vi "labview_camerasleft_hand_cameraimage_Server.vi"() -> ()   [LabVIEW 2013]
doc: "Template server that runs individual ros topics, services, etc. This is cloned for each topic being run."
uses:
  SubVIs/_ROSControl.ctl
  SubVIs/_ROSDirection.ctl
  _ROSDefinition.vi
panel:
  out "Init Count":i32
  out "queue":string
  out "Connected":bool
  out "str to write":string
  out "Status":T1(ring) caption="Connected?"
  out "Specs":T3={"Server"="", "Node"="/labview", "Server Port"=5000, "URI (Subsc)"="", "Direction"=enum."Node"}
  out "Service Reply":string
  out "unregister":string="<?xml version='1.0'?>\n<methodResponse>\n<params>\n<param>\n<value><array><data>\n<value><int>1</int></value>\n<value><string>Registered [/labview] as publisher of [/robot/head/command_head_nod]</string></value>\n<value><array><data>\n<value><string>http://tuftsBaxter.local:56995/</string></value>\n</data></array></value>\n</data></array></value>\n</param>\n</params>\n</methodResponse>\n"
  out "Requests":T4(array[cluster])
  out "Last Reply":string
  in  "stop":bool
  out "error out":errorcluster
  out "Connections":T5(array[cluster])
  in  "Baxter":T6
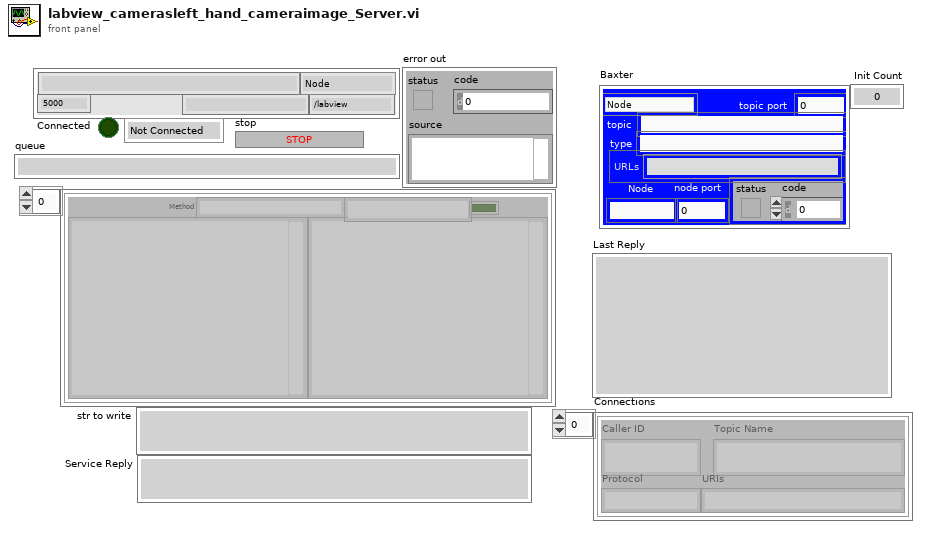
[diagram p1: front panel]
types:
  T1 = enum16{"Not Connected", "Registered", "Connected"}
  T2 = typedef "_ROSDirection.ctl" = enum16{"Node", "Publisher", "Subscriber", "Service Client"}
  T3 = cluster{"Server":string, "Node":string, "Server Port":u32, "URI (Subsc)":string, "Direction":T2}
  T4 = cluster{"First":string, "Second":string, "Method":string, "success":bool, "Dir1":string, "Dir2":string, "time":string}[]
  T5 = cluster{"Caller ID":string, "Topic Name":string, "Protocol":string, "URIs":string}[]
  T6 = typedef "_ROSControl.ctl" = cluster{"topic port":u16, "Node":string, "topic":string, "type":string, "node port":u32, "error ":errorcluster, "Direction":T2, "APIs":string[]}
  T7 = cluster{"data out":string, "data out 2":string, "data out 3":string, "Success?":bool, "data out 4":string, "data out 5":string, "time":string}[]
  T8 = cluster{"Code":i32, "Status Message":string, "APIs":string[]}
  T9 = cluster{"Server":string, "Node":string, "Server Port":u32, "URI (Subsc)":string, "connection":refnum<k5>, "Direction":T2}
  T10 = cluster{"Caller ID":string, "Topic Name":string, "Protocol":string, "URIs":string}
  T11 = cluster{string, "data out":string, "Node":string, bool, string, string, "Current Time":string}
  T12 = cluster{string, string, string, bool, string, string, "Current Time":string}
  T13 = cluster{"Protocol":string, "Code":i32, "IP":string, "Port":i32}
  T14 = cluster{"Node":string, "topic":string, "topic":string, "topic":string}
  T15 = cluster{"Code":i8, "statusMessage":string, "APIs":string[]}
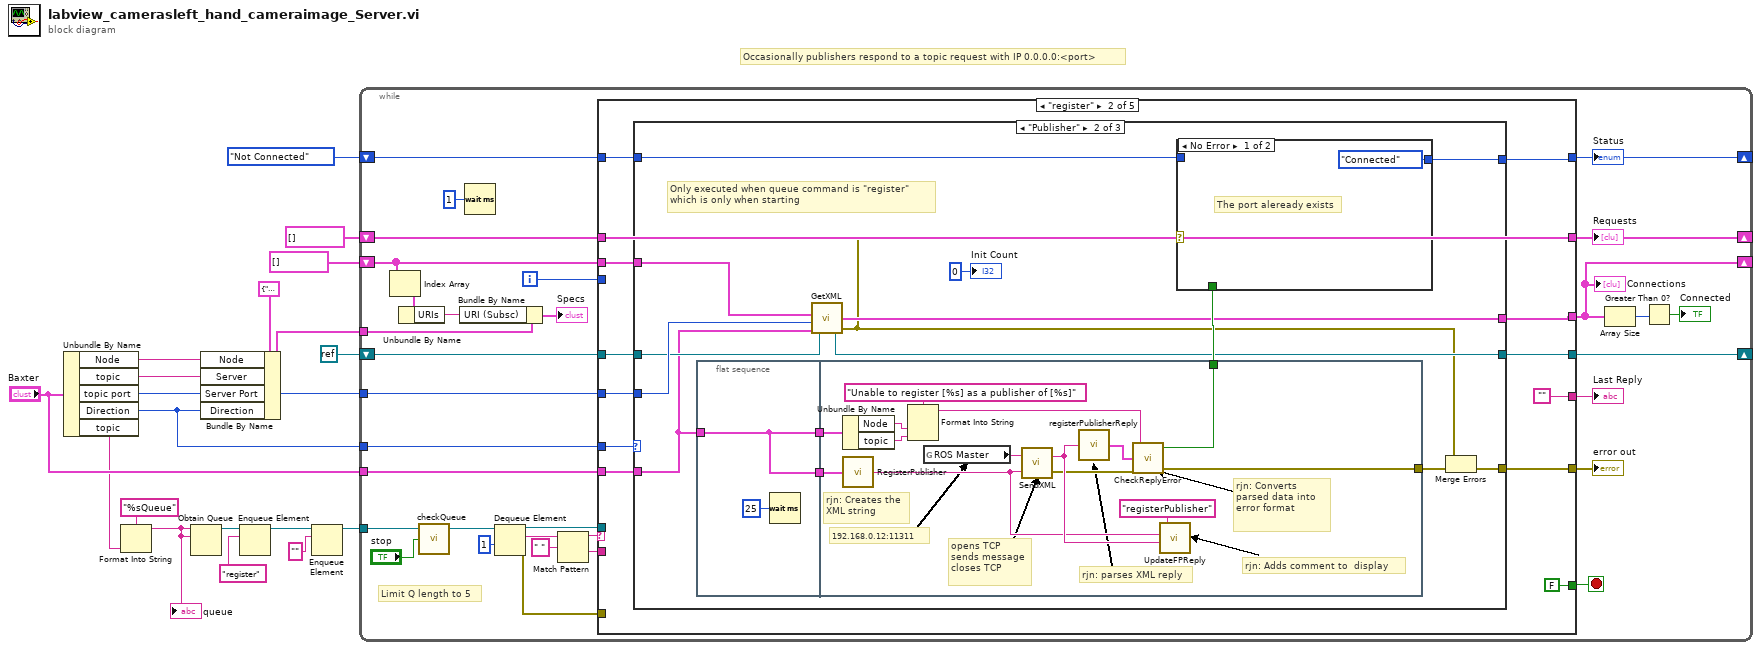
[diagram p0: block diagram]
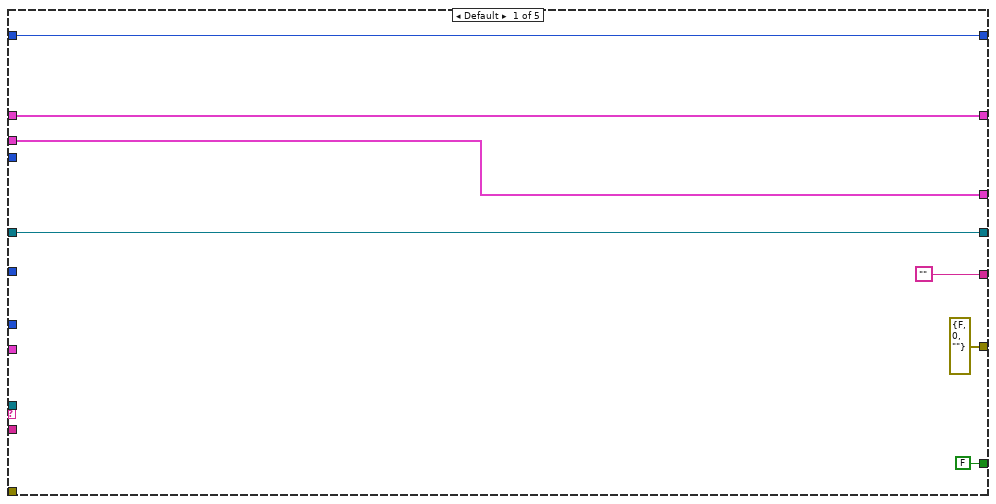
[diagram p2: hidden frame]
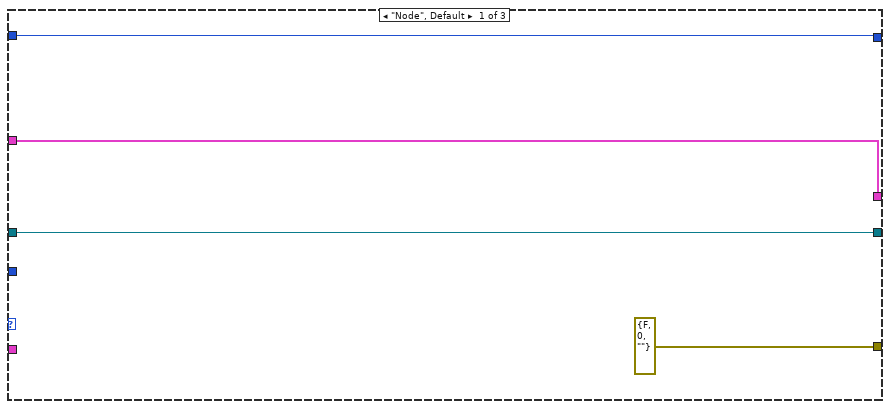
[diagram p3: hidden frame]
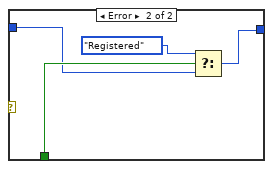
[diagram p4: hidden frame]
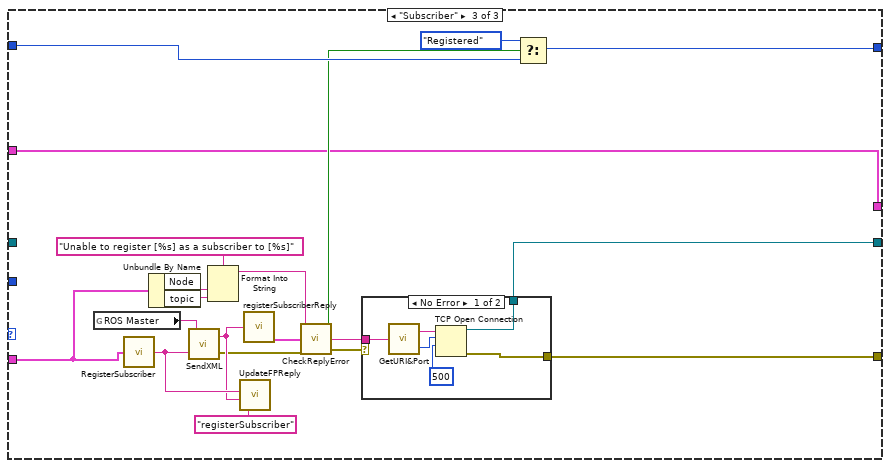
[diagram p5: hidden frame]
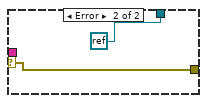
[diagram p6: hidden frame]
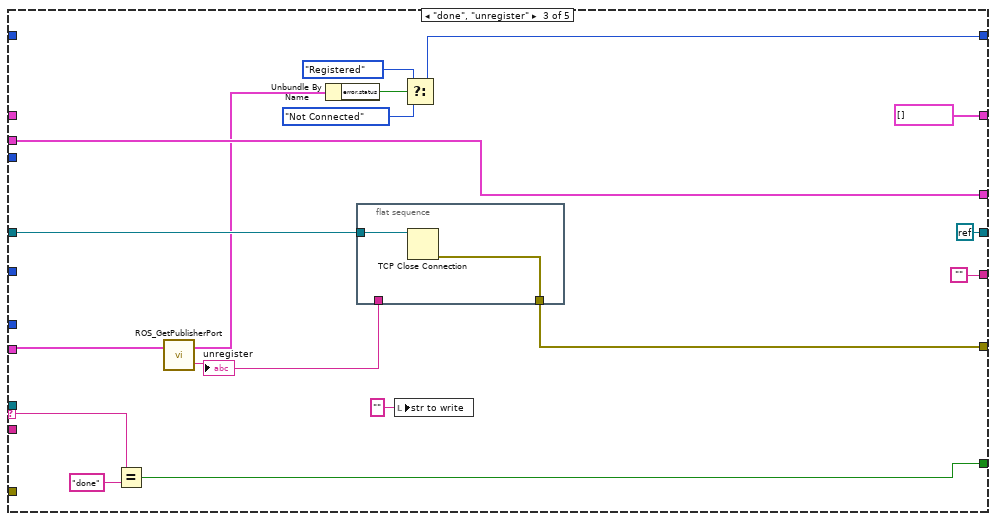
[diagram p7: hidden frame]
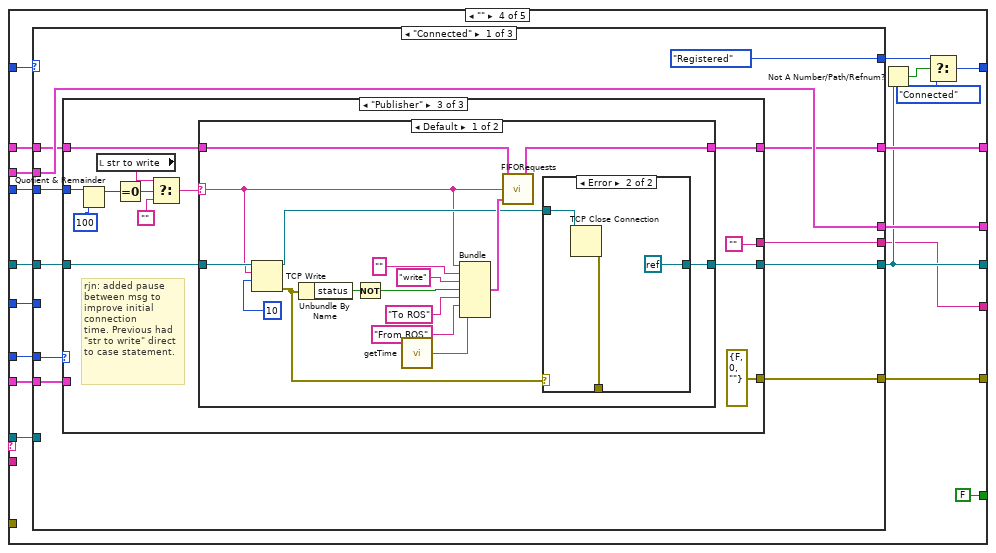
[diagram p8: hidden frame]
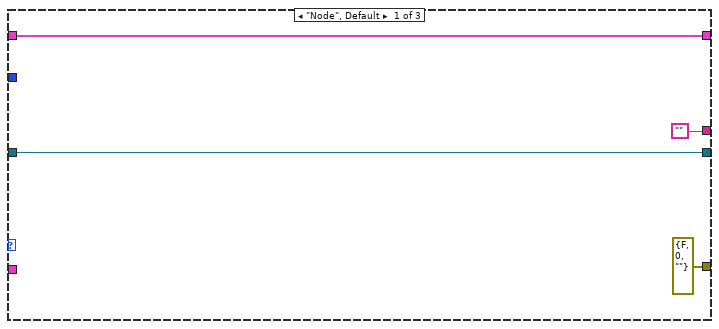
[diagram p9: hidden frame]
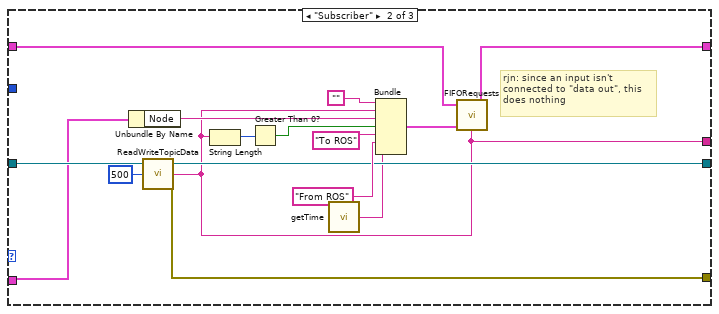
[diagram p10: hidden frame]
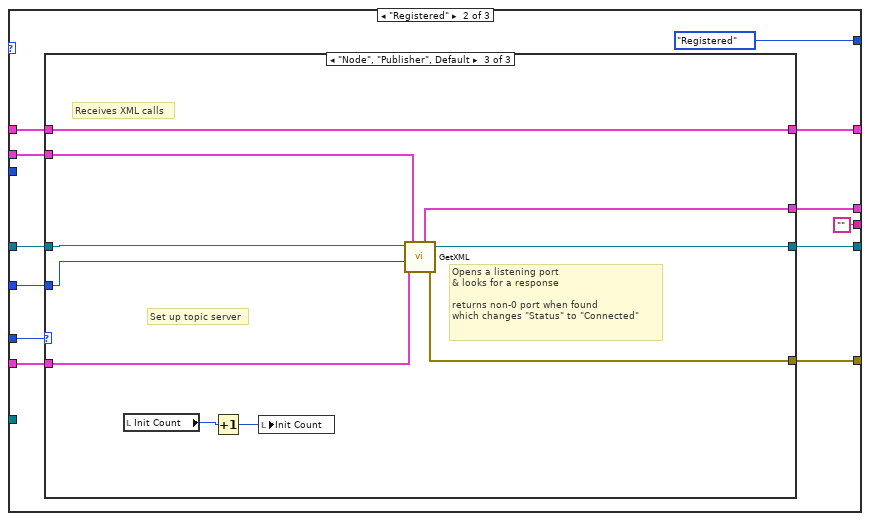
[diagram p13: hidden frame]
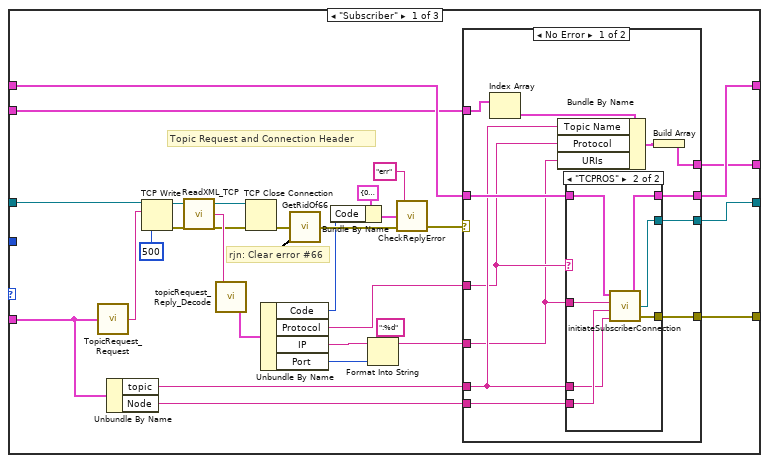
[diagram p14: hidden frame]
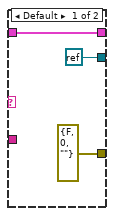
[diagram p15: hidden frame]
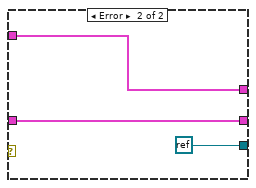
[diagram p16: hidden frame]
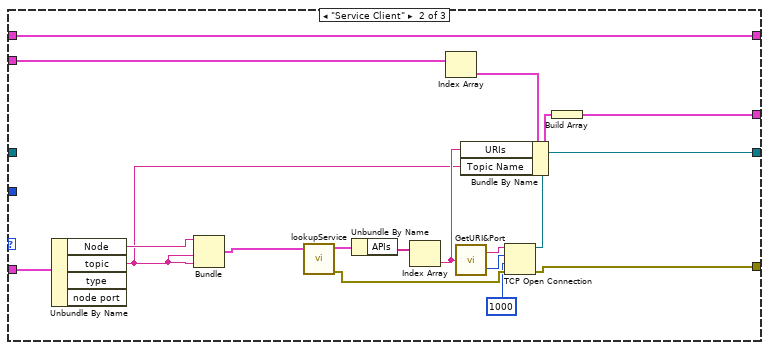
[diagram p17: hidden frame]
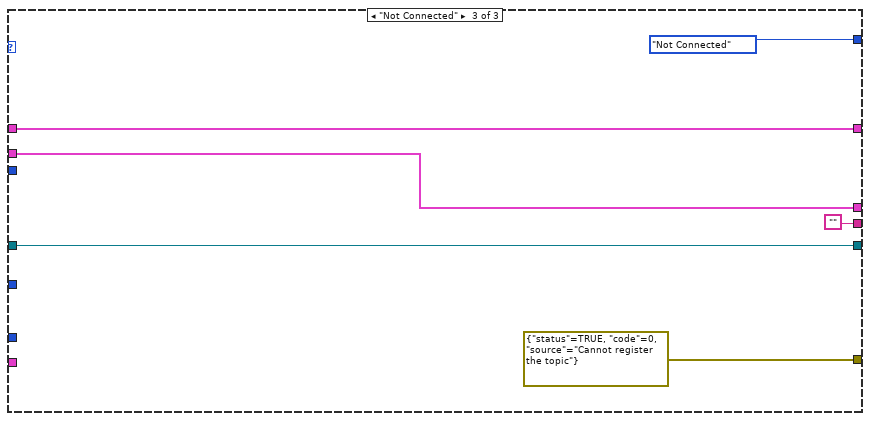
[diagram p18: hidden frame]
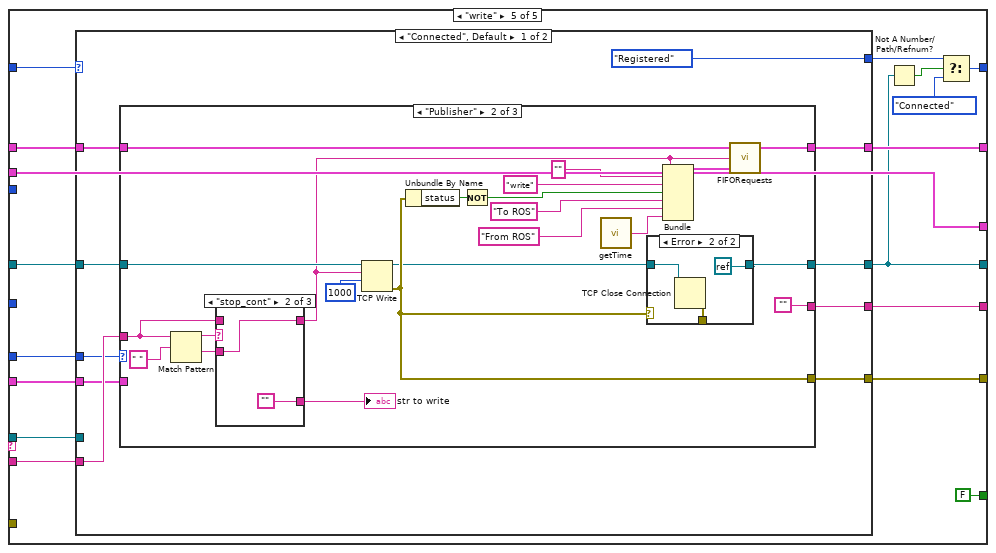
[diagram p19: hidden frame]
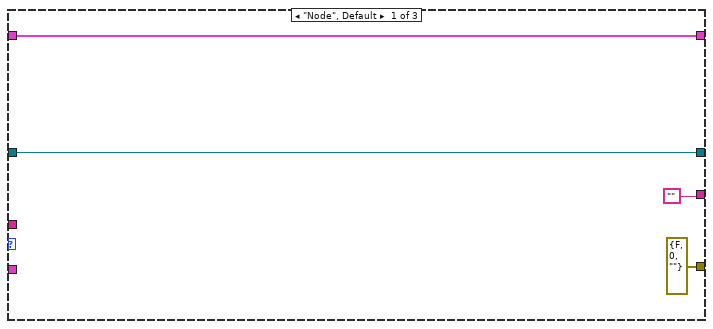
[diagram p20: hidden frame]
diagram:
  # "Occasionally publishers respond to a topic request with IP 0.0.0.0:<port>"
  n1 = Unbundle By Name("Baxter") -> ("Node"=w4:string, "topic"=w3:string, "topic port"=w1:u16, "Direction"=w2:T2, "topic"=w9:string)
  n2 = Format Into String(format string="%sQueue", w9) -> (resulting string=w18:string)  [unwired: 2 in, 1 out]
  "queue" <- w18
  n3 = Obtain Queue(name (unnamed)=w18, element data type=w18) -> (queue out=w12:refnum<queue>)  [unwired: 3 in, 2 out]
  n4 = Bundle By Name(cluster=T3 {"Server"="", "Node"="/labview", "Server Port"=5000, "URI (Subsc)"="", "Direction"=enum."Node"} ("Specs"), "Node"=w4, "Server"=w3, "Server Port"=w1, "Direction"=w2) -> (w10:T3)
  n5 = Enqueue Element(queue=w12, element="register") -> (queue out=w7:refnum<queue>)  [unwired: 2 in, 2 out]
  n6 = Enqueue Element(queue=w7, element="") -> (queue out=w6:refnum<queue>)  [unwired: 2 in, 2 out]
  n7 = while {
    tunnel: w1 -> [w51]
    shift-right: [w25] -> _
    shift-left: T5 [] ("Connections") -> [w34]
    shift-right: [w40] -> _
    shift-left: refnum<k0> refnum -> [w49]
    tunnel: w2 -> [w50]
    tunnel: "Baxter" -> [w48]
    shift-right: [w41] -> _
    shift-left: T7 [] ("Requests In") -> [w42]
    shift-right: [w37] -> _
    shift-left: T1."Not Connected" ("Status") -> [w38]
    tunnel: w10 -> [w32]
    tunnel: w6 -> [w26]
    i -> [w20]
    stop <- w39 stop-if-true
    # "Limit Q length to 5"
    n8 = Index Array(array=w34) -> (element=w33:T10)  [unwired: 1 in]
    n9 = Unbundle By Name(w33) -> ("URIs"=w31:string)
    n10 = call "checkQueue.vi"("stop"="stop", "queue in"=w26) -> ("queue out"=w28:refnum<queue>)  [unwired: 3 in]
    n11 = Bundle By Name(cluster=w32, "URI (Subsc)"=w31) -> (→"Specs":T3)
    n12 = Wait (ms)(milliseconds to wait=u32 1 ("millisecond multiple")) -> ()  [unwired: 1 out]
    n13 = Dequeue Element(queue=w28, timeout in ms (-1)=1) -> (queue out=w29:refnum<queue>, element=w46:string, error out=w22:errorcluster)  [unwired: 1 in, 1 out]
    n14 = Match Pattern(string=w46, regular expression=" ") -> (before substring=w44:string, after substring=w43:string)  [unwired: 1 in, 2 out]
    n15 = case shown="\"register\"" w44 {
      selector: w44 -> [_ _ w145 _ _]
      tunnel: w51 -> [_ w70 _ w177 _]
      tunnel: w34 -> [w58 w62 w155 w176 w361]
      tunnel: [w58 w61 w155 w175 w361] -> w25
      tunnel: w50 -> [_ w71 _ w174 w353]
      tunnel: [w57 w67 refnum<k0> refnum w168 w354] -> w40
      tunnel: w49 -> [w57 w66 w156 w169 w360]
      tunnel: w48 -> [_ w69 w154 w173 w351]
      tunnel: w43 -> [_ _ _ _ w358]
      tunnel: [FALSE FALSE w143 FALSE FALSE] -> w39
      tunnel: [errorcluster {"status"=FALSE, "code"=0, "source"=""} ("error out") w68 w148 w170 w355] -> w36
      tunnel: w42 -> [w56 w65 _ w172 w357]
      tunnel: [w56 w65 T7 [] ("Requests Out") w171 w356] -> w41
      tunnel: w38 -> [w55 w64 _ w162 w359]
      tunnel: [w55 w63 w150 w163 w346] -> w37
      tunnel: ["" "" "" w167 w352] -> w35
      tunnel: w29 -> [_ _ _ w166 w350]
      tunnel: w22 -> [_ _ _ _ _]
      tunnel: w20 -> [_ _ _ w159 _]
      frame Default {
      }
      frame "register" {
        n16 = case shown="\"Publisher\"" w71 {
          tunnel: w70 -> [_ w85 _]
          tunnel: w69 -> [_ w82 w122]
          tunnel: [errorcluster {"status"=FALSE, "code"=0, "source"=""} ("error IO") w80 w119] -> w68
          tunnel: [w75 w83 w120] -> w67
          tunnel: w66 -> [w75 w84 _]
          tunnel: w64 -> [w74 w89 w115]
          tunnel: [w74 w88 w113] -> w63
          tunnel: w62 -> [w73 w87 w112]
          tunnel: [w73 w86 w112] -> w61
          frame "Node", Default {
          }
          frame "Publisher" {
            # "Only executed when queue command is \"register\"\nwhich is only when starting"
            n17 = flat-sequence {
              tunnel: w82 -> [w91]
              tunnel: [w91] -> w78
              tunnel: [w91] -> w76
              tunnel: [w96] -> w90
              tunnel: [w94] -> w81
              tunnel: w78 -> [w95]
              tunnel: w76 -> [w93]
              frame #0 {
                n18 = Wait (ms)(milliseconds to wait=u32 25) -> ()  [unwired: 1 out]
              }
              frame #1 {
                # "rjn: Adds comment to  display"
                # "rjn: Converts parsed data into\nerror format"
                # "rjn: parses XML reply"
                # "192.168.0.12:11311"
                # "opens TCP\nsends message\ncloses TCP"
                # "rjn: Creates the \nXML string"
                n19 = Unbundle By Name(w95) -> ("Node"=w102:string, "topic"=w101:string)
                n20 = call "RegisterPublisher.vi"("ROS"=w93) -> ("XML"=w100:string)
                n21 = Format Into String(format string="Unable to register [%s] as a publisher of [%s]", w102, w101) -> (resulting string=w98:string)  [unwired: 2 in, 1 out]
                n22 = global read "_ROSDefinition.vi" "ROS Master"() -> (w106:string)
                n23 = call "SendXML.vi"("Send"=w100, "URI in"=w106) -> ("error out"=w97:errorcluster, "Reply"=w105:string)
                n24 = call "registerPublisherReply.vi"("Response"=w105) -> ("Response"=w99:T8)
                n25 = call "CheckReplyError.vi"("error in"=w97, "Response"=w99, "Error String"=w98) -> ("error out"=w94:errorcluster, "Registered?"=w96:bool)  [unwired: 1 out]
                n26 = call "UpdateFPReply.vi"("Reply"=w105, "Sent"=w100, "method"="registerPublisher") -> ()  [unwired: 3 in]
              }
            }
            n27 = call "GetXML.vi"("Baxter"=w82, "topic port"=w85, "Connections"=w87, "connection ID in"=w84) -> ("error IO"=w79:errorcluster, "Subscribers"=w86:T5, "connection ID out"=w83:refnum<k5>)
            n28 = case shown="No Error" w79 {
              tunnel: w90 -> [_ w111]
              tunnel: w89 -> [_ w110]
              tunnel: [T1."Connected" ("f") w108] -> w88
              frame No Error {
                # "The port aleready exists"
              }
              frame Error {
                n29 = Select(t=T1."Registered", s=w111, f=w110) -> (s? t:f=w108:T1)
              }
            }
            n30 = Merge Errors(w79, w81) -> (w80:errorcluster)
            "Init Count" <- 0
          }
          frame "Subscriber" {
            n31 = global read "_ROSDefinition.vi" "ROS Master"() -> (w131:string)
            n32 = call "RegisterSubscriber.vi"("ROS"=w122) -> ("XML"=w129:string)
            n33 = Unbundle By Name(w122) -> ("Node"=w126:string, "topic"=w125:string)
            n34 = call "SendXML.vi"("Send"=w129, "URI in"=w131) -> ("error out"=w118:errorcluster, "Reply"=w128:string)
            n35 = Format Into String(format string="Unable to register [%s] as a subscriber to [%s]", w126, w125) -> (resulting string=w123:string)  [unwired: 2 in, 1 out]
            n36 = call "UpdateFPReply.vi"("Reply"=w128, "Sent"=w129, "method"="registerSubscriber") -> ()  [unwired: 3 in]
            n37 = call "registerSubscriberReply.vi"("Response"=w128) -> ("Response"=w127:T8)
            n38 = call "CheckReplyError.vi"("error in"=w118, "Response"=w127, "Error String"=w123) -> ("error out"=w117:errorcluster, "URI"=w121:string, "Registered?"=w114:bool)
            n39 = case shown="No Error" w117 {
              selector: w117 -> [_ w139]
              tunnel: w121 -> [w137 _]
              tunnel: [w133 refnum<k0> refnum] -> w120
              tunnel: [w132 w139] -> w119
              frame No Error {
                n40 = call "GetURI&Port.vi"("URI in"=w137) -> ("Port"=w135:u16, "URI"=w136:string)
                n41 = TCP Open Connection(address=w136, remote port or service name=w135, timeout ms (60000)=500) -> (connection ID=w133:refnum<k5>, error out=w132:errorcluster)  [unwired: 2 in]
              }
              frame Error {
              }
            }
            n42 = Select(t=T1."Registered", s=w114, f=w115) -> (s? t:f=w113:T1)
          }
        }
      }
      frame "done", "unregister" {
        n43 = Equal?(x=w145, y="done") -> (x = y?=w143:bool)
        n44 = call "ROS_GetPublisherPort.vi"("ROS in"=w154) -> ("Response"=w146:string, "ROS out"=w153:T6)  [unwired: 1 in]
        "unregister" <- w146
        n45 = Unbundle By Name(w153) -> ("error.status"=w149:bool)
        n46 = flat-sequence {
          tunnel: w156 -> [w158]
          tunnel: [w157] -> w148
          tunnel: w146 -> [_]
          frame #0 {
            n47 = TCP Close Connection(connection ID=w158) -> (error out=w157:errorcluster)  [unwired: 2 in, 1 out]
          }
        }
        n48 = local write "str to write"("" ("str to write")) -> ()
        n49 = Select(t=T1."Registered" ("Status"), s=w149, f=T1."Not Connected") -> (s? t:f=w150:T1)
      }
      frame "" {
        n50 = case shown="\"Connected\"" w162 {
          tunnel: w177 -> [_ w255 _]
          tunnel: w176 -> [w187 w254 w343]
          tunnel: [w187 w253 w343] -> w175
          tunnel: w174 -> [w188 w252 _]
          tunnel: [w181 w251 w342] -> w168
          tunnel: w169 -> [w186 w250 w342]
          tunnel: w173 -> [w185 w249 _]
          tunnel: w172 -> [w184 w248 w344]
          tunnel: [w183 w247 w344] -> w171
          tunnel: [w182 w246 errorcluster {"status"=TRUE, "code"=0, "source"="Cannot register the topic"} ("error out")] -> w170
          tunnel: [w180 "" ""] -> w167
          tunnel: w166 -> [_ _ _]
          tunnel: [T1."Registered" ("f") T1."Registered" ("f") T1."Not Connected" ("f")] -> w161
          tunnel: w159 -> [w178 _ _]
          frame "Connected" {
            n51 = case shown="\"Publisher\"" w188 {
              tunnel: w186 -> [w191 w208 w219]
              tunnel: w185 -> [_ w201 _]
              tunnel: w184 -> [w192 w206 w221]
              tunnel: [w192 w205 w220] -> w183
              tunnel: [errorcluster {"status"=FALSE, "code"=0, "source"=""} ("error out") w204 errorcluster {"status"=FALSE, "code"=0, "source"=""} ("error out")] -> w182
              tunnel: [w191 w195 w218] -> w181
              tunnel: ["" w194 ""] -> w180
              tunnel: w178 -> [_ _ w215]
              frame "Node", Default {
              }
              frame "Subscriber" {
                # "rjn: since an input isn't\nconnected to \"data out\", this\ndoes nothing"
                n52 = Unbundle By Name(w201) -> ("Node"=w200:string)
                n53 = call "ReadWriteTopicData.vi"("timeout ms (1000)"=500, "connection ID in"=w208) -> ("error out"=w204:errorcluster, "data out"=w194:string, "connection ID out"=w195:refnum<k5>)  [unwired: 1 in]
                n54 = String Length(string=w194) -> (length=w203:i32)
                n55 = Greater Than 0?(x=w203) -> (x > 0?=w199:bool)
                n56 = call "getTime.vi"() -> ("Current Time"=w193:string)  [unwired: 1 in]
                n57 = Bundle("", "data out"=w194, "Node"=w200, w199, "To ROS", "From ROS", "Current Time"=w193) -> (w196:T11)  [unwired: 1 in]
                n58 = call "FIFORequests.vi"("New One"=w196, "data out"=w194, "Requests In"=w206) -> ("Requests Out"=w205:T7)
              }
              frame "Publisher" {
                # "rjn: added pause \nbetween msg to \nimprove initial\nconnection\ntime. Previous had\n\"str to write\" direct\nto case statement."
                n59 = Quotient & Remainder(x=w215, y=100) -> (x-y*floor(x/y)=w213:i32)  [unwired: 1 out]
                n60 = local read "str to write"() -> (w211:string)
                n61 = Equal To 0?(x=w213) -> (x = 0?=w212:bool)
                n62 = Select(t=w211, s=w212, f="") -> (s? t:f=w209:string)
                n63 = case shown="Default" w209 {
                  selector: w209 -> [w222 _]
                  tunnel: w221 -> [w230 w243]
                  tunnel: [w229 w243] -> w220
                  tunnel: w219 -> [w227 w242]
                  tunnel: [w226 w242] -> w218
                  frame Default {
                    n64 = TCP Write(connection ID=w227, data in=w222, 9:10 ("timeout ms (25000)")) -> (connection ID out=w231:refnum<k5>, error out=w225:errorcluster)  [unwired: 1 in, 1 out]
                    n65 = Unbundle By Name(w225) -> ("status"=w233:bool)
                    n66 = Not(x=w233) -> (.not. x?=w232:bool)
                    n67 = call "getTime.vi"() -> ("Current Time"=w223:string)  [unwired: 1 in]
                    n68 = Bundle(w222, "", "write", w232, "To ROS", "From ROS", "Current Time"=w223) -> (w234:T12)  [unwired: 1 in]
                    n69 = call "FIFORequests.vi"("New One"=w234, "data out"=w222, "Requests In"=w230) -> ("Requests Out"=w229:T7)
                    n70 = case shown="Error" w225 {
                      tunnel: w231 -> [w238 w241]
                      tunnel: [w238 refnum<k0> refnum] -> w226
                      tunnel: [_ w239] -> _
                      frame No Error {
                      }
                      frame Error {
                        n71 = TCP Close Connection(connection ID=w241) -> (error out=w239:errorcluster)  [unwired: 2 in, 1 out]
                      }
                    }
                  }
                  frame "" {
                  }
                }
              }
            }
          }
          frame "Registered" {
            n72 = case shown="\"Node\", \"Publisher\", Default" w252 {
              tunnel: w255 -> [_ _ w331]
              tunnel: w254 -> [w265 w316 w338]
              tunnel: [w264 w314 w337] -> w253
              tunnel: [w268 w320 w336] -> w251
              tunnel: w250 -> [w285 _ w332]
              tunnel: w249 -> [w273 w327 w335]
              tunnel: w248 -> [w271 w328 w334]
              tunnel: [w270 w328 w334] -> w247
              tunnel: [w269 w319 w333] -> w246
              frame "Subscriber" {
                # "rjn: Clear error #66"
                # "Topic Request and Connection Header"
                n73 = call "TopicRequest_Request.vi"("ROS"=w273) -> ("XML"=w284:string)
                n74 = Unbundle By Name(w273) -> ("topic"=w256:string, "Node"=w272:string)
                n75 = TCP Write(connection ID=w285, data in=w284, 9:500 ("timeout ms (25000)")) -> (connection ID out=w283:refnum<k5>, error out=w282:errorcluster)  [unwired: 1 in, 1 out]
                n76 = call "ReadXML_TCP.vi"("error in"=w282, "connection ID in"=w283) -> ("error out"=w278:errorcluster, "data out"=w280:string, "connection ID out"=w279:refnum<k5>)  [unwired: 1 in]
                n77 = call "topicRequest_Reply_Decode.vi"("Topic Request Reply"=w280) -> ("Topic Request Reply"=w277:T13)
                n78 = TCP Close Connection(connection ID=w279, error in (no error)=w278) -> (error out=w276:errorcluster)  [unwired: 1 in, 1 out]
                n79 = Unbundle By Name(w277) -> ("Code"=w259:i32, "Protocol"=w267:string, "IP"=w263:string, "Port"=w274:i32)
                n80 = call "GetRidOf66.vi"("error in (no error)"=w276) -> ("error out"=w261:errorcluster)
                n81 = Bundle By Name(cluster=T8 {"Code"=0, "Status Message"="", "APIs"=[]} ("Response"), "Code"=w259) -> (w257:T8)
                n82 = Format Into String(format string=":%d", initial string=w263, w274) -> (resulting string=w266:string)  [unwired: 1 in, 1 out]
                n83 = call "CheckReplyError.vi"("error in"=w261, "Response"=w257, "Error String"="err" ("source")) -> ("error out"=w260:errorcluster)  [unwired: 2 out]
                n84 = case shown="No Error" w260 {
                  tunnel: w267 -> [w289 _]
                  tunnel: w266 -> [w288 _]
                  tunnel: w272 -> [w297 _]
                  tunnel: w256 -> [w290 _]
                  tunnel: w271 -> [w296 w308]
                  tunnel: [w295 w308] -> w270
                  tunnel: [w294 _] -> w269
                  tunnel: [w293 refnum<k0> refnum] -> w268
                  tunnel: w265 -> [w292 w309]
                  tunnel: [w286 w309] -> w264
                  frame No Error {
                    n85 = Index Array(array=w292) -> (element=w291:T10)  [unwired: 1 in]
                    n86 = Bundle By Name(cluster=w291, "Topic Name"=w290, "Protocol"=w289, "URIs"=w288) -> (w287:T10)
                    n87 = case shown="\"TCPROS\"" w289 {
                      tunnel: w288 -> [_ w307]
                      tunnel: w297 -> [_ w306]
                      tunnel: w290 -> [_ w305]
                      tunnel: w296 -> [w299 w301]
                      tunnel: [w299 w304] -> w295
                      tunnel: [errorcluster {"status"=FALSE, "code"=0, "source"=""} ("error out") w303] -> w294
                      tunnel: [refnum<k0> refnum w302] -> w293
                      frame Default {
                      }
                      frame "TCPROS" {
                        n88 = call "initiateSubscriberConnection.vi"("topic"=w305, "Node"=w306, "URI"=w307, "Requests In"=w301) -> ("error out"=w303:errorcluster, "connection ID out"=w302:refnum<k5>, "Requests Out"=w304:T7)
                      }
                    }
                    n89 = Build Array(w287) -> (w286:T5)
                  }
                  frame Error {
                  }
                }
              }
              frame "Service Client" {
                n90 = Unbundle By Name(w327) -> ("Node"=w326:string, "topic"=w312:string)  [unwired: 2 out]
                n91 = Bundle("Node"=w326, "topic"=w312, "topic"=w312, "topic"=w312) -> (w325:T14)  [unwired: 1 in]
                n92 = call "lookupService.vi"("Parameters"=w325) -> ("Reply"=w324:T15, "error out"=w313:errorcluster)  [unwired: 4 in, 2 out]
                n93 = Unbundle By Name(w324) -> ("APIs"=w323:string[])
                n94 = Index Array(array=w323) -> (element=w317:string)  [unwired: 1 in]
                n95 = Index Array(array=w316) -> (element=w318:T10)  [unwired: 1 in]
                n96 = call "GetURI&Port.vi"("URI in"=w317) -> ("Port"=w321:u16, "URI"=w322:string)
                n97 = Bundle By Name(cluster=w318, "URIs"=w317, "Topic Name"=w312) -> (w315:T10)
                n98 = TCP Open Connection(address=w322, remote port or service name=w321, timeout ms (60000)=1000, error in (no error)=w313) -> (connection ID=w320:refnum<k5>, error out=w319:errorcluster)  [unwired: 1 in]
                n99 = Build Array(w315) -> (w314:T5)
              }
              frame "Node", "Publisher", Default {
                # "Opens a listening port\n& looks for a response\n\nreturns non-0 port when found\nwhich changes \"Status\" to \"Connected\""
                # "Set up topic server"
                # "Receives XML calls"
                n100 = local read "Init Count"() -> (w330:i32)
                n101 = Increment(x=w330) -> (x+1=w329:i32)
                n102 = local write "Init Count"(w329) -> ()
                n103 = call "GetXML.vi"("Baxter"=w335, "topic port"=w331, "Connections"=w338, "connection ID in"=w332) -> ("error IO"=w333:errorcluster, "Subscribers"=w337:T5, "connection ID out"=w336:refnum<k5>)
              }
            }
          }
          frame "Not Connected" {
          }
        }
        n104 = Not A Number/Path/Refnum?(number/path/refnum=w168) -> (NaN/Path/Refnum?=w164:bool)
        n105 = Select(t=w161, s=w164, f=T1."Connected") -> (s? t:f=w163:T1)
      }
      frame "write" {
        n106 = case shown="\"Connected\", Default" w359 {
          tunnel: w360 -> [w371 w430]
          tunnel: w358 -> [w368 w427]
          tunnel: w357 -> [w370 w431]
          tunnel: [w369 w431] -> w356
          tunnel: [w366 w430] -> w354
          tunnel: [w367 errorcluster {"status"=FALSE, "code"=0, "source"=""} ("error out")] -> w355
          tunnel: w353 -> [w365 _]
          tunnel: [w364 ""] -> w352
          tunnel: w351 -> [w363 _]
          tunnel: w350 -> [_ w429]
          tunnel: [T1."Registered" ("f") T1."Connected" ("f")] -> w347
          frame "Connected", Default {
            n107 = case shown="\"Publisher\"" w365 {
              tunnel: w371 -> [w374 w397 w413]
              tunnel: w370 -> [w375 w395 w422]
              tunnel: [w375 w394 w421] -> w369
              tunnel: w368 -> [_ w378 w420]
              tunnel: [errorcluster {"status"=FALSE, "code"=0, "source"=""} ("error out") w386 w419] -> w367
              tunnel: [w374 w384 refnum<k0> refnum] -> w366
              tunnel: ["" "" w418] -> w364
              tunnel: w363 -> [_ _ w417]
              frame "Node", Default {
              }
              frame "Publisher" {
                n108 = Match Pattern(string=w378, regular expression=" ") -> (before substring=w379:string, after substring=w380:string)  [unwired: 1 in, 2 out]
                n109 = case shown="\"stop_cont\"" w379 {
                  tunnel: w380 -> [_ w401 w402]
                  tunnel: [w398 w401 w402] -> w382
                  tunnel: ["" "" w402] -> w381
                  tunnel: w378 -> [w398 _ _]
                  frame Default {
                  }
                  frame "stop_cont" {
                  }
                  frame "cont" {
                  }
                }
                "str to write" <- w381
                n110 = TCP Write(connection ID=w397, data in=w382, 9:1000 ("timeout ms (25000)")) -> (connection ID out=w385:refnum<k5>, error out=w386:errorcluster)  [unwired: 1 in, 1 out]
                n111 = Unbundle By Name(w386) -> ("status"=w388:bool)
                n112 = Not(x=w388) -> (.not. x?=w387:bool)
                n113 = call "getTime.vi"() -> ("Current Time"=w377:string)  [unwired: 1 in]
                n114 = case shown="Error" w386 {
                  tunnel: w385 -> [w403 w406]
                  tunnel: [w403 refnum<k0> refnum] -> w384
                  tunnel: [_ w404] -> _
                  frame No Error {
                  }
                  frame Error {
                    n115 = TCP Close Connection(connection ID=w406) -> (error out=w404:errorcluster)  [unwired: 2 in, 1 out]
                  }
                }
                n116 = Bundle(w382, "", "write", w387, "To ROS", "From ROS", "Current Time"=w377) -> (w389:T12)  [unwired: 1 in]
                n117 = call "FIFORequests.vi"("New One"=w389, "data out"=w382, "Requests In"=w395) -> ("Requests Out"=w394:T7)
              }
              frame "Service Client" {
                n118 = Unbundle By Name(w417) -> ("topic"=w409:string, "Node"=w410:string, "APIs"=w415:string[], "Direction"=w408:T2)
                n119 = Index Array(array=w415) -> (element=w414:string)  [unwired: 1 in]
                n120 = local write "Service Reply"("" ("Service Reply")) -> ()
                n121 = Bundle By Name(cluster=T9 {"Server"="", "Node"="/labview", "Server Port"=5000, "URI (Subsc)"="", "connection"=refnum, "Direction"=enum."Node"} ("Specs"), "Server"=w409, "Node"=w410, "URI (Subsc)"=w414, "connection"=w413, "Direction"=w408) -> (w412:T9)
                n122 = call "ROS_Service_Setup.vi"("Specs"=w412, "Msg to Send"=w420, "Requests In"=w422) -> ("error out"=w419:errorcluster, "Reply"=w418:string, "Requests Out"=w421:T7)
                "Service Reply" <- w418
              }
            }
          }
          frame "Not Connected" {
            n123 = Format Into String(format string="write %s", w427) -> (resulting string=w426:string)  [unwired: 2 in, 1 out]
            n124 = call "cleanQueue.vi"("String"=w426, "queue in"=w429) -> ()  [unwired: 1 in, 1 out]
          }
        }
        n125 = Not A Number/Path/Refnum?(number/path/refnum=w354) -> (NaN/Path/Refnum?=w348:bool)
        n126 = Select(t=w347, s=w348, f=T1."Connected") -> (s? t:f=w346:T1)
      }
    }
    "error out" <- w36
    "Requests" <- w41
    "Status" <- w37
    "Connections" <- w25
    "Last Reply" <- w35
    n127 = Array Size(array=w25) -> (size(s)=w24:i32)
    n128 = Greater Than 0?(x=w24) -> (x > 0?=→"Connected":bool)
  }
